vi "main.vi"() -> ()   [LabVIEW 2014]
uses:
  Step/Control/Step name enum.ctl
  Controls/Step array.ctl
  Controls/INI config.ctl
  <vilib>/DAQmx/read.llb/DAQmx Read (Analog DBL 1Chan 1Samp).vi
  <vilib>/Automated Test Systems Ltd/General Tools/Que lib/Initialise.vi
  <vilib>/Automated Test Systems Ltd/General Tools/Que lib/Write.vi
  <vilib>/DAQmx/miscellaneous.llb/DAQmx Fill In Error Info.vi
  Controls/ResultsGlobal.vi
  Controls/ConditionsGlobal.vi
  <vilib>/DAQmx/create/channels.llb/DAQmx Create Channel (AI-Temperature-Thermocouple).vi
  Step/Step global.vi
  Step/Test status global.vi
  <vilib>/Instr/_visa.llb/VISA Configure Serial Port (Instr).vi
  <vilib>/Automated Test Systems Ltd/Device drivers/SensorMetrix/Lib/Read T3110.vi
  <vilib>/NI/Modbus Library/API/Master/Modbus Master.lvclass
  <vilib>/Automated Test Systems Ltd/General Tools/Que lib/Que lib.lvlib
  <vilib>/Automated Test Systems Ltd/General Tools/Stopwatch/Stop watch/Stop watch.lvlib
  <vilib>/Automated Test Systems Ltd/Device drivers/SensorMetrix/Lib/T3110 & T2114.lvlib
panel:
  out "Test Status":string[](array[string])
  out "T3110 Temperature":dbl
  out "NI Temperature":dbl
  out "Arduino Temperature":dbl
  out "Step elapsed time, ms":u32
  out "Test elapsed time, ms":u32
  in  "pause":bool
  in  "abort":bool
  out "Step cluster":T2={"Step number"=0, "Step Name"="", "Step name enum"=enum."Init NI", "Start condition 1 name"="", "Start condition 1 comparator"="", "Start condition 1 value"=0.0, "Start condition 2 name"="", "Start condition 2 comparator"="", "Start condition 2 value"=0.0, "Start condition 3 name"="", "Start condition 3 comparator"="", "Start condition 3 value"=0.0, "End condition 1 name"="", "End condition 1 comparator"="", "End condition 1 value"=0.0, "End condition 2 name"="", "End condition 2 comparator"="", "End condition 2 value"=0.0, "End condition 3 name"="", "End condition 3 comparator"="", "End condition 3 value"=0.0, "Constant condition 1 name"="", "Constant condition 1 comparator"="", "Constant condition 1 value"=0.0, "Constant condition 2 name"="", "Constant condition 2 comparator"="", "Constant condition 2 value"=0.0, "Constant condition 3 name"="", "Constant condition 3 comparator"="", "Constant condition 3 value"=0.0, "Duration"=0.0, "Max Duration"=0.0}
  out "Test running":bool
  in  "file path (dialog if empty)":path
  in  "Start profile":bool
  out "Test profile INI":string[][](array[string])
  in  "stop":bool
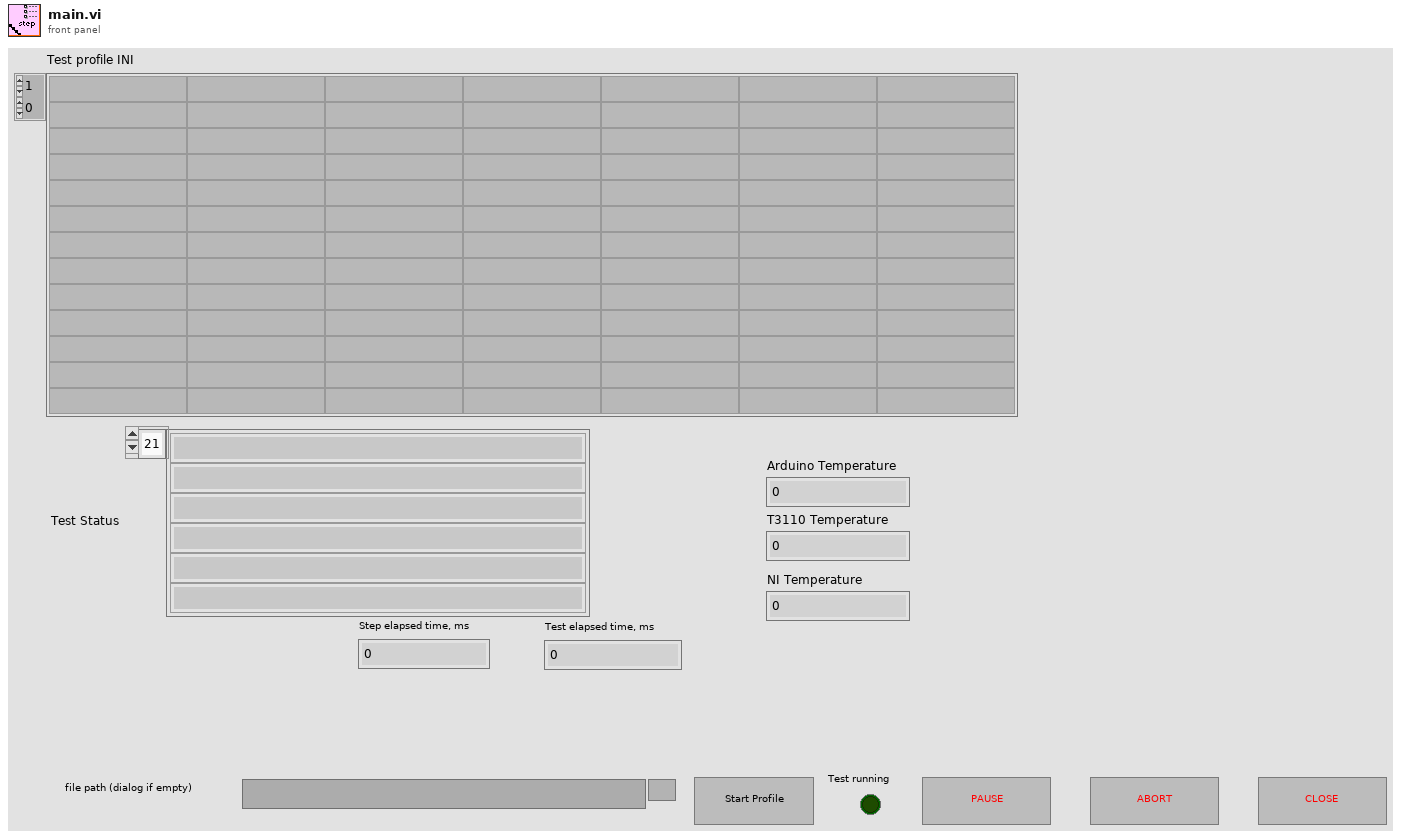
[diagram p1: front panel]
types:
  T1 = typedef "Step name enum.ctl" = enum16{"Default", "Idle", "Init Ard", "Init SM", "Init NI", "Run", "Close"}
  T2 = cluster{"Step number":i32, "Step Name":string, "Step name enum":T1, "Start condition 1 name":string, "Start condition 1 comparator":string, "Start condition 1 value":dbl, "Start condition 2 name":string, "Start condition 2 comparator":string, "Start condition 2 value":dbl, "Start condition 3 name":string, "Start condition 3 comparator":string, "Start condition 3 value":dbl, "End condition 1 name":string, "End condition 1 comparator":string, "End condition 1 value":dbl, "End condition 2 name":string, "End condition 2 comparator":string, "End condition 2 value":dbl, "End condition 3 name":string, "End condition 3 comparator":string, "End condition 3 value":dbl, "Constant condition 1 name":string, "Constant condition 1 comparator":string, "Constant condition 1 value":dbl, "Constant condition 2 name":string, "Constant condition 2 comparator":string, "Constant condition 2 value":dbl, "Constant condition 3 name":string, "Constant condition 3 comparator":string, "Constant condition 3 value":dbl, "Duration":dbl, "Max Duration":dbl}
  T3 = typedef "INI config.ctl" = cluster{"Config":cluster{"DAQ channel":string, "T3110 COM":string, "Arduino COM":string}, "Parameters":cluster{"Max temp":dbl, "Min temp":dbl}}
  T4 = typedef "Step array.ctl" = cluster{"Step number":i32, "Step Name":string, "Step name enum":T1, "Start condition 1 name":string, "Start condition 1 comparator":string, "Start condition 1 value":dbl, "Start condition 2 name":string, "Start condition 2 comparator":string, "Start condition 2 value":dbl, "Start condition 3 name":string, "Start condition 3 comparator":string, "Start condition 3 value":dbl, "End condition 1 name":string, "End condition 1 comparator":string, "End condition 1 value":dbl, "End condition 2 name":string, "End condition 2 comparator":string, "End condition 2 value":dbl, "End condition 3 name":string, "End condition 3 comparator":string, "End condition 3 value":dbl, "Constant condition 1 name":string, "Constant condition 1 comparator":string, "Constant condition 1 value":dbl, "Constant condition 2 name":string, "Constant condition 2 comparator":string, "Constant condition 2 value":dbl, "Constant condition 3 name":string, "Constant condition 3 comparator":string, "Constant condition 3 value":dbl, "Duration, mS":dbl, "Max Duration, mS":dbl}[]
  T5 = cluster{"Step number":i32, "Step Name":string, "Step name enum":T1, "Start condition 1 name":string, "Start condition 1 comparator":string, "Start condition 1 value":dbl, "Start condition 2 name":string, "Start condition 2 comparator":string, "Start condition 2 value":dbl, "Start condition 3 name":string, "Start condition 3 comparator":string, "Start condition 3 value":dbl, "End condition 1 name":string, "End condition 1 comparator":string, "End condition 1 value":dbl, "End condition 2 name":string, "End condition 2 comparator":string, "End condition 2 value":dbl, "End condition 3 name":string, "End condition 3 comparator":string, "End condition 3 value":dbl, "Constant condition 1 name":string, "Constant condition 1 comparator":string, "Constant condition 1 value":dbl, "Constant condition 2 name":string, "Constant condition 2 comparator":string, "Constant condition 2 value":dbl, "Constant condition 3 name":string, "Constant condition 3 comparator":string, "Constant condition 3 value":dbl, "Duration, mS":dbl, "Max Duration, mS":dbl}
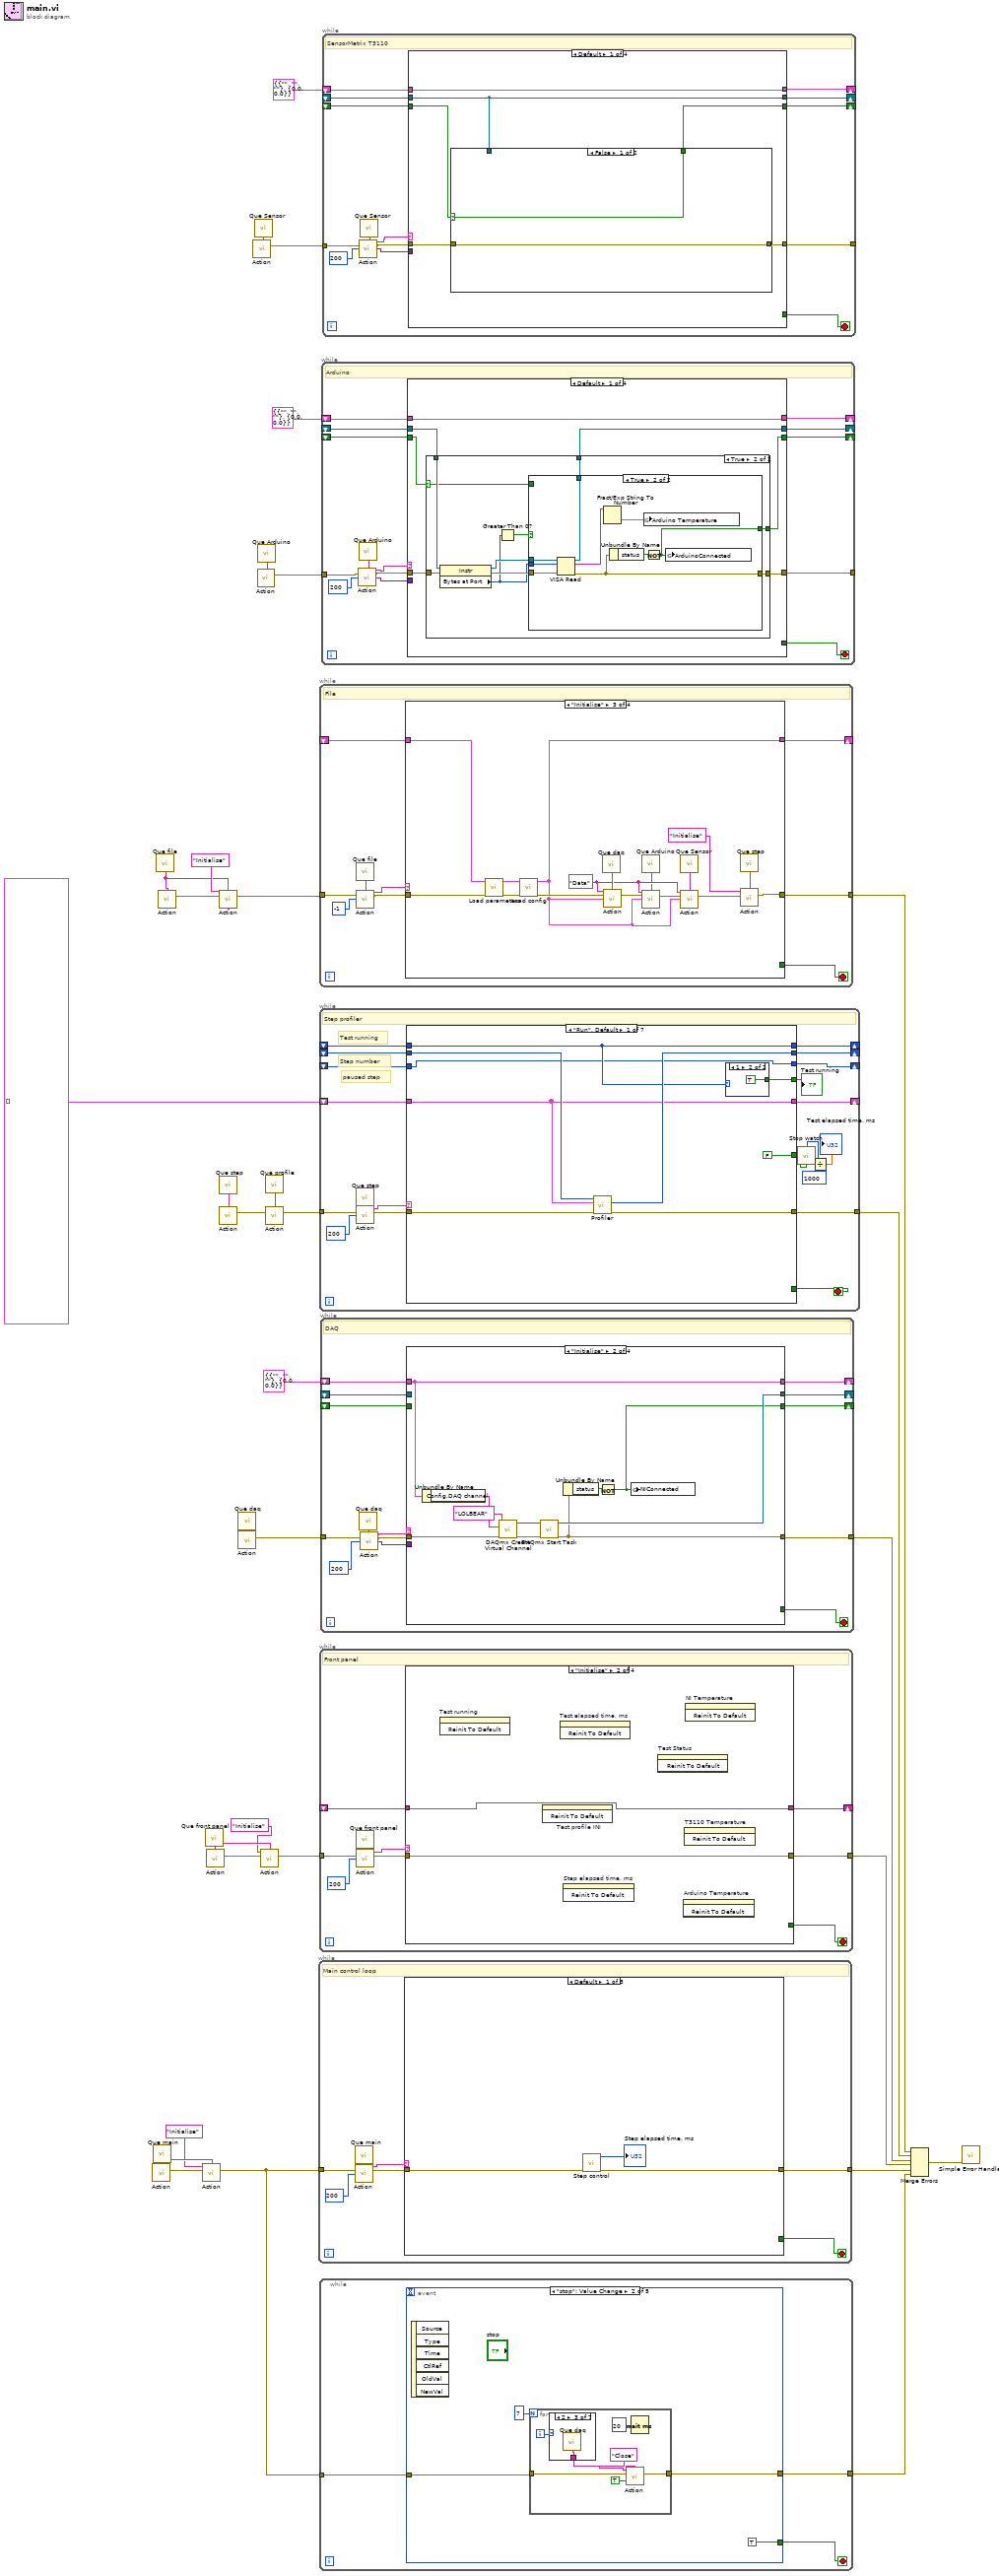
[diagram p0: block diagram]
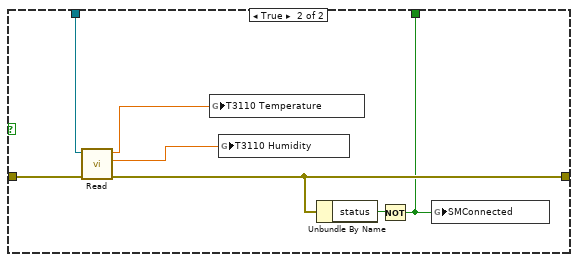
[diagram p2: hidden frame]
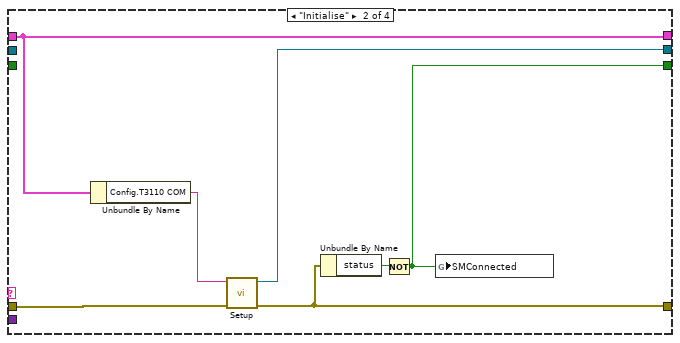
[diagram p3: hidden frame]
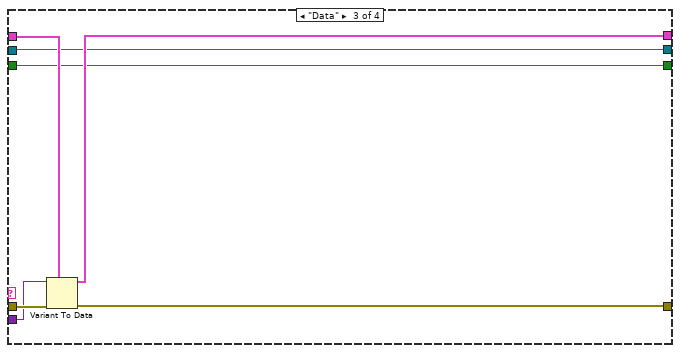
[diagram p4: hidden frame]
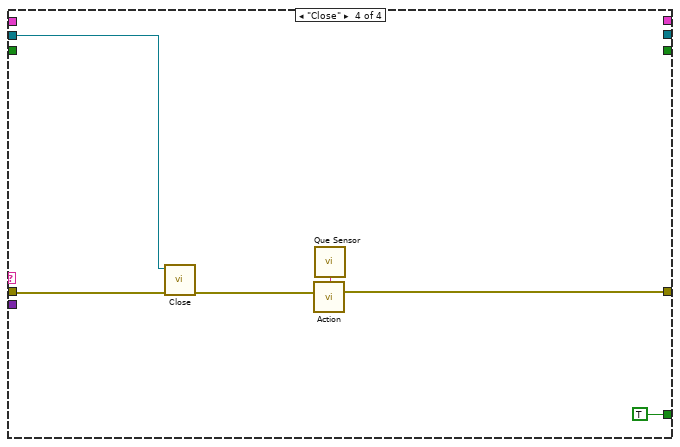
[diagram p5: hidden frame]
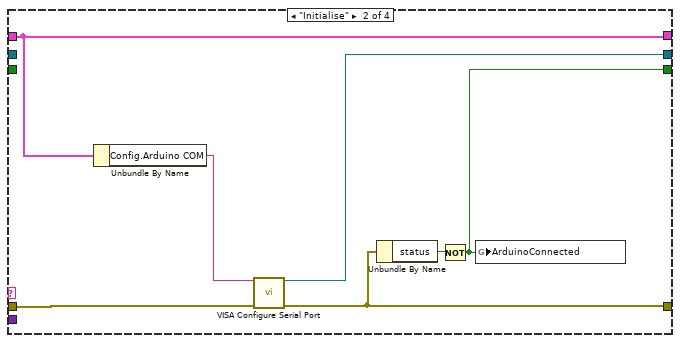
[diagram p8: hidden frame]
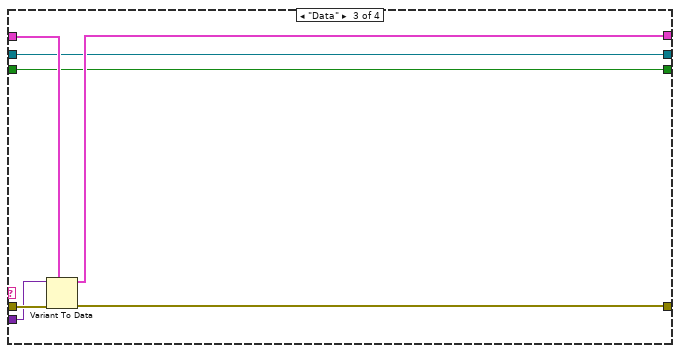
[diagram p9: hidden frame]
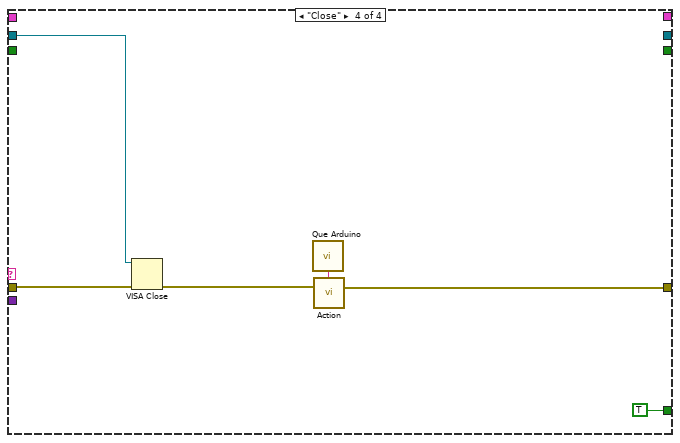
[diagram p10: hidden frame]
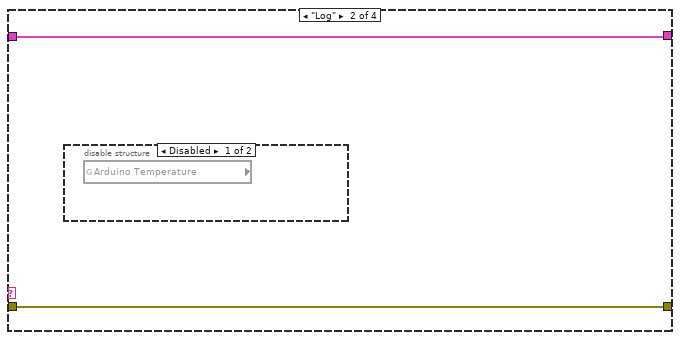
[diagram p12: hidden frame]
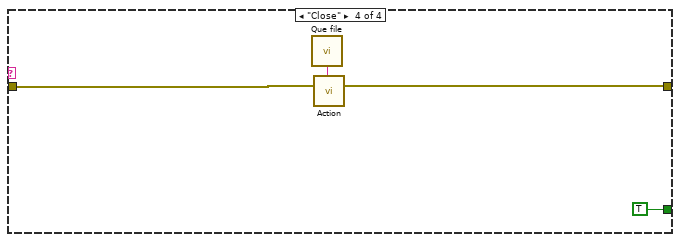
[diagram p14: hidden frame]
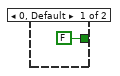
[diagram p15: hidden frame]
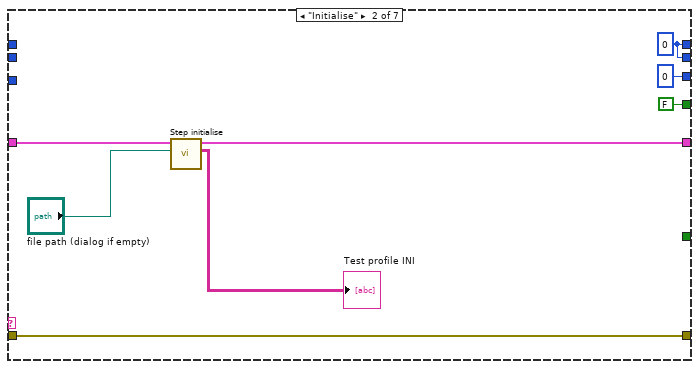
[diagram p16: hidden frame]
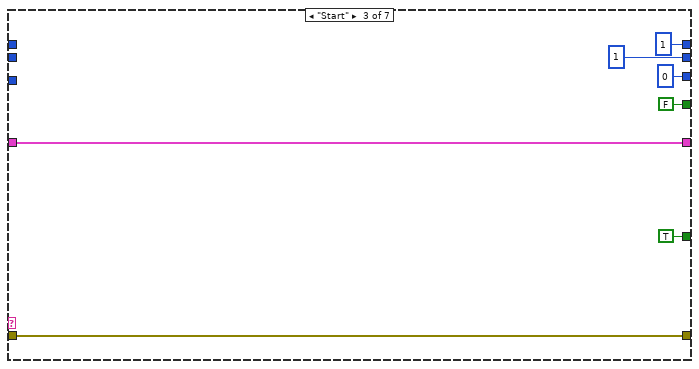
[diagram p17: hidden frame]
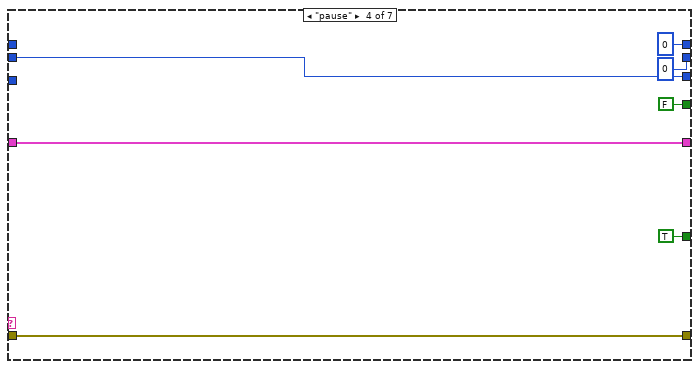
[diagram p18: hidden frame]
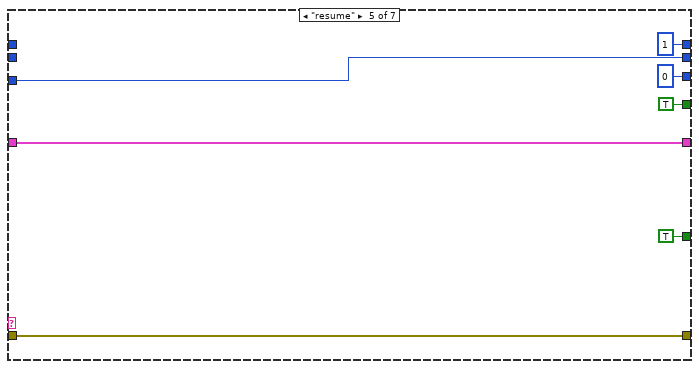
[diagram p19: hidden frame]
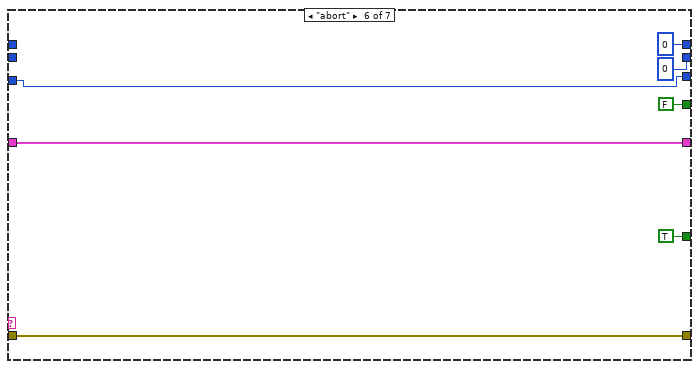
[diagram p20: hidden frame]
diagram:
  n1 = call <vilib>:"Que main.vi"() -> ("Que name"=w10:string)  [unwired: 15 in]
  n2 = call-poly <vilib>:"Action.vi"("Que name"=w10) -> ("error out"=w11:errorcluster)  [unwired: 14 in]
  n3 = call <vilib>:"Que file.vi"() -> ("Que name"=w22:string)  [unwired: 15 in]
  n4 = call-poly <vilib>:"Action.vi"("Que name"=w22) -> ("error out"=w23:errorcluster)  [unwired: 14 in]
  n5 = call-poly <vilib>:"Action.vi"("Message"="Initialise" ("Command"), "Que name"=w10, "error in"=w11) -> ("error out"=w8:errorcluster)  [unwired: 12 in]
  n6 = call <vilib>:"Que front panel.vi"() -> ("Que name"=w14:string)  [unwired: 15 in]
  n7 = call-poly <vilib>:"Action.vi"("Que name"=w14) -> ("error out"=w15:errorcluster)  [unwired: 14 in]
  n8 = call-poly <vilib>:"Action.vi"("Message"="Initialise" ("Command"), "Que name"=w22, "error in"=w23) -> ("error out"=w24:errorcluster)  [unwired: 12 in]
  n9 = call <vilib>:"Que step.vi"() -> ("Que name"=w18:string)  [unwired: 15 in]
  n10 = call-poly <vilib>:"Action.vi"("Que name"=w18) -> ("error out"=w21:errorcluster)  [unwired: 14 in]
  n11 = call <vilib>:"Que daq.vi"() -> ("Que name"=w17:string)  [unwired: 15 in]
  n12 = call-poly <vilib>:"Action.vi"("Que name"=w17) -> ("error out"=w16:errorcluster)  [unwired: 14 in]
  n13 = call <vilib>:"Que Sensor.vi"() -> ("Que name"=w4:string)  [unwired: 15 in]
  n14 = call-poly <vilib>:"Action.vi"("Que name"=w4) -> ("error out"=w3:errorcluster)  [unwired: 14 in]
  n15 = call <vilib>:"Que Arduino.vi"() -> ("Que name"=w6:string)  [unwired: 15 in]
  n16 = call-poly <vilib>:"Action.vi"("Que name"=w6) -> ("error out"=w7:errorcluster)  [unwired: 14 in]
  n17 = call-poly <vilib>:"Action.vi"("Message"="Initialise" ("Command"), "Que name"=w14, "error in"=w15) -> ("error out"=w13:errorcluster)  [unwired: 12 in]
  n18 = call <vilib>:"Que profile.vi"() -> ("Que name"=w19:string)  [unwired: 15 in]
  n19 = call-poly <vilib>:"Action.vi"("Que name"=w19, "error in"=w21) -> ("error out"=w20:errorcluster)  [unwired: 13 in]
  n20 = while {
    tunnel: w8 -> [w36]
    tunnel: [w40] -> w32
    stop <- w39 stop-if-true
    # "Main control loop"
    n21 = call <vilib>:"Que main.vi"() -> ("Que name"=w38:string)  [unwired: 15 in]
    n22 = call-poly <vilib>:"Action.vi"("Que name"=w38, "error in"=w36, "Timeout (default 2s)"=200 ("Timeout")) -> ("Message out"=w34:string, "error out"=w37:errorcluster)  [unwired: 10 in, 1 out]
    n23 = case shown="Default" w34 {
      tunnel: w37 -> [w43 w44 w46]
      tunnel: [w42 w44 w47] -> w40
      tunnel: [_ _ TRUE] -> w39
      frame Default {
        n24 = call "Step control.vi"("error in"=w43) -> ("error out"=w42:errorcluster, "Step elapsed time,  s"=→"Step elapsed time, ms":u32)  [unwired: 9 in]
      }
      frame "Initialise" {
      }
      frame "Close" {
        n25 = call <vilib>:"Que main.vi"() -> ("Que name"=w45:string)  [unwired: 15 in]
        n26 = call-poly <vilib>:"Action.vi"("Que name"=w45, "error in"=w46) -> ("error out"=w47:errorcluster)  [unwired: 13 in]
      }
    }
  }
  n27 = while {
    tunnel: w20 -> [w53]
    tunnel: [w67] -> w29
    shift-right: [w65] -> _
    shift-left: T4 [] ("Step array") -> [w66]
    shift-right: [w64] -> _
    shift-left: _ -> [w63]
    shift-right: [w61] -> _
    shift-left: _ -> [w62]
    shift-right: [w58] -> _
    shift-left: _ -> [w59]
    stop <- w68 stop-if-true
    # "paused step"
    # "Step number"
    # "Test running"
    # "Step profiler"
    n28 = call <vilib>:"Que step.vi"() -> ("Que name"=w51:string)  [unwired: 15 in]
    n29 = call-poly <vilib>:"Action.vi"("Que name"=w51, "error in"=w53, "Timeout (default 2s)"=200 ("Timeout")) -> ("Message out"=w54:string, "error out"=w55:errorcluster)  [unwired: 10 in, 1 out]
    n30 = case shown="\"Run\", Default" w54 {
      tunnel: w55 -> [w73 w87 w92 w99 w105 w112 w117]
      tunnel: [_ _ _ _ _ _ TRUE] -> w68
      tunnel: [w74 w87 w92 w99 w105 w112 w118] -> w67
      tunnel: w66 -> [w75 w85 w93 w96 w104 w113 w123]
      tunnel: [w75 w83 w93 w96 w104 w113 w123] -> w65
      tunnel: [w72 w86 1 0 1 0 0] -> w64
      tunnel: w63 -> [w72 _ _ _ _ _ _]
      tunnel: w62 -> [w77 _ _ w98 _ _ _]
      tunnel: [w76 w86 1 0 ("Step number") w107 0 ("Step number") 0] -> w61
      tunnel: [w70 FALSE FALSE FALSE TRUE FALSE FALSE] -> w60
      tunnel: w59 -> [w71 _ _ _ w107 w110 _]
      tunnel: [w71 0 ("Step number") 0 ("Step number") w98 0 ("Step number") w110 0 ("Step number")] -> w58
      tunnel: [FALSE _ TRUE TRUE TRUE TRUE _] -> w49
      frame "Run", Default {
        n31 = call "Profiler.vi"("error in"=w73, "Step array"=w75, "Step number"=w77) -> ("error out"=w74:errorcluster, "Step number"=w76:i32)  [unwired: 6 in, 1 out]
        n32 = case shown="1" w72 {
          tunnel: [FALSE TRUE] -> w70
          frame 0, Default {
          }
          frame 1 {
          }
        }
      }
      frame "Initialise" {
        w86 = 0
        n33 = call "Step initialise.vi"("file path (dialog if empty)"="file path (dialog if empty)", "Step array"=w85) -> ("all rows"=→"Test profile INI":string[][], "Step array out"=w83:T4)  [unwired: 8 in]
      }
      frame "Start" {
      }
      frame "pause" {
      }
      frame "resume" {
      }
      frame "abort" {
      }
      frame "Close" {
        n34 = call <vilib>:"Que step.vi"() -> ("Que name"=w116:string)  [unwired: 15 in]
        n35 = call-poly <vilib>:"Action.vi"("Que name"=w116, "error in"=w117) -> ("error out"=w118:errorcluster)  [unwired: 13 in]
      }
    }
    "Test running" <- w60
    n36 = call <vilib>:"Stop watch.vi"("reset timer"=w49) -> ("Elapsed time, ms"=w50:u32)  [unwired: 13 in, 1 out]
    n37 = Divide(x=w50, y=1000) -> (x/y=→"Test elapsed time, ms":dbl)
  }
  n38 = while {
    tunnel: w13 -> [w127]
    tunnel: [w132] -> w31
    shift-right: [w131] -> _
    shift-left: _ -> [w130]
    stop <- w133 stop-if-true
    # "Front panel"
    n39 = call <vilib>:"Que front panel.vi"() -> ("Que name"=w129:string)  [unwired: 15 in]
    n40 = call-poly <vilib>:"Action.vi"("Que name"=w129, "error in"=w127, "Timeout (default 2s)"=200 ("Timeout")) -> ("Message out"=w126:string, "error out"=w128:errorcluster)  [unwired: 10 in, 1 out]
    n41 = case shown="\"Initialise\"" w126 {
      tunnel: w128 -> [w142 w144 w146 w151]
      tunnel: [_ _ _ TRUE] -> w133
      tunnel: [w142 w144 w146 w148] -> w132
      tunnel: [w135 w143 w145 w150] -> w131
      tunnel: w130 -> [w140 w143 w145 w150]
      frame Default {
        n42 = global read "Step global.vi" "Step cluster"() -> (w141:T5)
        "Step cluster" <- w141
        n43 = global read "Test status global.vi" "Test status"() -> (w139:string)
        n44 = Unbundle(w141) -> ()  [unwired: 32 out]
        n45 = call <vilib>:"FILO string equal.vi"("Array"=w140, "Array size"=200, "String"=w139) -> ("Array out"=w135:string[])  [unwired: 12 in]
        "Test Status" <- w135
        n46 = global read "ResultsGlobal.vi" "Arduino Temperature"() -> (→"Arduino Temperature":dbl)
        n47 = global read "ResultsGlobal.vi" "T3110 Temperature"() -> (→"T3110 Temperature":dbl)
        n48 = global read "ResultsGlobal.vi" "NI Temperature"() -> (→"NI Temperature":dbl)
      }
      frame "Initialise" {
        n49 = invoke on="Test running" class="Bool (strict)" method="Reinit To Default"() -> ()  [unwired: 3 in, 3 out]
        n50 = invoke on="Test profile INI" class="Arr (strict)" method="Reinit To Default"() -> ()  [unwired: 3 in, 3 out]
        n51 = invoke on="Test elapsed time, ms" class="DigNum (strict)" method="Reinit To Default"() -> ()  [unwired: 3 in, 3 out]
        n52 = invoke on="Step elapsed time, ms" class="DigNum (strict)" method="Reinit To Default"() -> ()  [unwired: 3 in, 3 out]
        n53 = invoke on="Test Status" class="Arr (strict)" method="Reinit To Default"() -> ()  [unwired: 3 in, 3 out]
        n54 = invoke on="Arduino Temperature" class="DigNum (strict)" method="Reinit To Default"() -> ()  [unwired: 3 in, 3 out]
        n55 = invoke on="T3110 Temperature" class="DigNum (strict)" method="Reinit To Default"() -> ()  [unwired: 3 in, 3 out]
        n56 = invoke on="NI Temperature" class="DigNum (strict)" method="Reinit To Default"() -> ()  [unwired: 3 in, 3 out]
      }
      frame "clear" {
      }
      frame "Close" {
        n57 = invoke on="Test profile INI" class="Arr (strict)" method="Reinit To Default"(error in=w151) -> (error out=w149:errorcluster)  [unwired: 2 in, 2 out]
        n58 = call <vilib>:"Que front panel.vi"() -> ("Que name"=w147:string)  [unwired: 15 in]
        n59 = call-poly <vilib>:"Action.vi"("Que name"=w147, "error in"=w149) -> ("error out"=w148:errorcluster)  [unwired: 13 in]
      }
    }
  }
  n60 = while {
    tunnel: w8 -> [w155]
    tunnel: [w154] -> w33
    stop <- w153 stop-if-true
    n61 = event shown="[1] \"stop\": Value Change" {
      selector: _ -> [_ _ _ _ _]
      dyn-events: _ -> [_ _ _ _ _]
      timeout: _ -> [_ _ _ _ _]
      tunnel: w155 -> [_ w158 w176 w180 w184]
      tunnel: [_ w157 w178 w181 w185] -> w154
      tunnel: [_ TRUE _ _ _] -> w153
      event Timeout {
        n62 = event-data() -> ()  [unwired: 1 in, 2 out]
      }
      event "stop": Value Change {
        n63 = event-data() -> ()  [unwired: 1 in, 6 out]
        n64 = for {
          N: 7 -> [_]
          tunnel: w158 -> [w162]
          tunnel: [w163] -> w157
          i -> [w166]
          n65 = case shown="2" w166 {
            tunnel: [w167 w168 w169 w170 w171 w172 w173] -> w160
            frame 0, Default {
              n66 = call <vilib>:"Que file.vi"() -> ("Que name"=w167:string)  [unwired: 15 in]
            }
            frame 1 {
              n67 = call <vilib>:"Que front panel.vi"() -> ("Que name"=w168:string)  [unwired: 15 in]
            }
            frame 2 {
              n68 = call <vilib>:"Que daq.vi"() -> ("Que name"=w169:string)  [unwired: 15 in]
            }
            frame 3 {
              n69 = call <vilib>:"Que main.vi"() -> ("Que name"=w170:string)  [unwired: 15 in]
            }
            frame 4 {
              n70 = call <vilib>:"Que step.vi"() -> ("Que name"=w171:string)  [unwired: 15 in]
            }
            frame 5 {
              n71 = call <vilib>:"Que Arduino.vi"() -> ("Que name"=w172:string)  [unwired: 15 in]
            }
            frame 6 {
              n72 = call <vilib>:"Que Sensor.vi"() -> ("Que name"=w173:string)  [unwired: 15 in]
            }
          }
          n73 = call-poly <vilib>:"Action.vi"("Message"="Close" ("Command"), "Que name"=w160, "error in"=w162, "Priority message?"=TRUE) -> ("error out"=w163:errorcluster)  [unwired: 11 in]
          n74 = Wait (ms)(milliseconds to wait=u32 20) -> ()  [unwired: 1 out]
        }
      }
      event "abort": Value Change {
        n75 = event-data() -> ()  [unwired: 1 in, 6 out]
        n76 = call <vilib>:"Que step.vi"() -> ("Que name"=w177:string)  [unwired: 15 in]
        n77 = call-poly <vilib>:"Action.vi"("Message"="abort" ("Command"), "Que name"=w177, "error in"=w176, "Priority message?"=TRUE) -> ("error out"=w178:errorcluster)  [unwired: 11 in]
      }
      event "Start profile": Value Change {
        n78 = event-data() -> ()  [unwired: 1 in, 6 out]
        n79 = call <vilib>:"Que step.vi"() -> ("Que name"=w182:string)  [unwired: 15 in]
        n80 = call-poly <vilib>:"Action.vi"("Message"="Start" ("Command"), "Que name"=w182, "error in"=w180) -> ("error out"=w181:errorcluster)  [unwired: 12 in]
      }
      event "pause": Value Change {
        n81 = event-data() -> ()  [unwired: 1 in, 6 out]
        n82 = case shown="False" "pause" {
          tunnel: ["resume" ("Command") "pause" ("Command")] -> w183
          tunnel: ["PAUSE" ("Command") "RESUME" ("Command")] -> w187
          frame False {
          }
          frame True {
          }
        }
        n83 = property on="pause" class="Bool (strict)"("BoolText.Text"=w187) -> ()  [unwired: 2 in, 2 out]
        n84 = call <vilib>:"Que step.vi"() -> ("Que name"=w186:string)  [unwired: 15 in]
        n85 = call-poly <vilib>:"Action.vi"("Message"=w183, "Que name"=w186, "error in"=w184) -> ("error out"=w185:errorcluster)  [unwired: 12 in]
      }
    }
  }
  n86 = while {
    tunnel: w24 -> [w199]
    tunnel: [w200] -> w28
    shift-right: [w194] -> _
    shift-left: _ -> [w193]
    stop <- w201 stop-if-true
    # "File"
    n87 = call <vilib>:"Que file.vi"() -> ("Que name"=w195:string)  [unwired: 15 in]
    n88 = call-poly <vilib>:"Action.vi"("Que name"=w195, "error in"=w199, "Timeout (default 2s)"=-1 ("Timeout")) -> ("Message out"=w197:string, "error out"=w198:errorcluster)  [unwired: 10 in, 1 out]
    n89 = case shown="\"Initialise\"" w197 {
      tunnel: w198 -> [w203 w205 w218 w224]
      tunnel: [_ _ _ TRUE] -> w201
      tunnel: [w203 w205 w221 w223] -> w200
      tunnel: [w202 w204 w211 _] -> w194
      tunnel: w193 -> [w202 w204 w214 _]
      frame Default {
      }
      frame "Log" {
        n90 = disable-structure shown="Disabled" {
          frame Disabled {
            n91 = global read "ResultsGlobal.vi" "Arduino Temperature"() -> ()  [unwired: 1 out]
          }
          frame Enabled {
          }
        }
      }
      frame "Initialise" {
        w210 = "Data" ("Command")
        n92 = call "Load parameters.vi"("error in"=w218, "INI data"=w214) -> ("error out"=w217:errorcluster, "INI data out"=w215:T3)  [unwired: 8 in]
        n93 = call "Load config.vi"("error in"=w217, "INI data"=w215) -> ("error out"=w216:errorcluster, "INI data out"=w211:T3)  [unwired: 8 in]
        n94 = call <vilib>:"Que daq.vi"() -> ("Que name"=w219:string)  [unwired: 15 in]
        n95 = call-poly <vilib>:"Action.vi"("Message"=w210, "Que name"=w219, "error in"=w216, "Data"=w211) -> ("error out"=w213:errorcluster)  [unwired: 11 in]
        n96 = call <vilib>:"Que Arduino.vi"() -> ("Que name"=w208:string)  [unwired: 15 in]
        n97 = call-poly <vilib>:"Action.vi"("Message"=w210, "Que name"=w208, "error in"=w213, "Data"=w211) -> ("error out"=w212:errorcluster)  [unwired: 11 in]
        n98 = call <vilib>:"Que Sensor.vi"() -> ("Que name"=w209:string)  [unwired: 15 in]
        n99 = call-poly <vilib>:"Action.vi"("Message"=w210, "Que name"=w209, "error in"=w212, "Data"=w211) -> ("error out"=w207:errorcluster)  [unwired: 11 in]
        n100 = call <vilib>:"Que step.vi"() -> ("Que name"=w220:string)  [unwired: 15 in]
        n101 = call-poly <vilib>:"Action.vi"("Message"="Initialise" ("Command"), "Que name"=w220, "error in"=w207) -> ("error out"=w221:errorcluster)  [unwired: 12 in]
      }
      frame "Close" {
        n102 = call <vilib>:"Que file.vi"() -> ("Que name"=w222:string)  [unwired: 15 in]
        n103 = call-poly <vilib>:"Action.vi"("Que name"=w222, "error in"=w224) -> ("error out"=w223:errorcluster)  [unwired: 13 in]
      }
    }
  }
  n104 = while {
    tunnel: w16 -> [w236]
    tunnel: [w238] -> w30
    shift-right: [w231] -> _
    shift-left: T3 {"Config"={"DAQ channel"="", "T3110 COM"="", "Arduino COM"=""}, "Parameters"={"Max temp"=0.0, "Min temp"=0.0}} ("INI data") -> [w230]
    shift-right: [w229] -> _
    shift-left: _ -> [w228]
    shift-right: [w227] -> _
    shift-left: _ -> [w226]
    stop <- w239 stop-if-true
    # "DAQ"
    n105 = call <vilib>:"Que daq.vi"() -> ("Que name"=w237:string)  [unwired: 15 in]
    n106 = call-poly <vilib>:"Action.vi"("Que name"=w237, "error in"=w236, "Timeout (default 2s)"=200 ("Timeout")) -> ("Message out"=w234:string, "error out"=w235:errorcluster, "Data"=w232:variant)  [unwired: 10 in]
    n107 = case shown="\"Initialise\"" w234 {
      tunnel: w235 -> [w244 w259 w271 w274]
      tunnel: [_ _ _ TRUE] -> w239
      tunnel: [w243 w258 w267 w278] -> w238
      tunnel: w232 -> [_ _ w270 _]
      tunnel: w230 -> [w245 w260 w269 _]
      tunnel: [w245 w260 w268 _] -> w231
      tunnel: [w242 w261 w266 _] -> w229
      tunnel: w228 -> [w242 _ w266 w272]
      tunnel: [w240 w256 w265 _] -> w227
      tunnel: w226 -> [w241 _ w265 _]
      frame Default {
        n108 = case shown="True" w241 {
          selector: w241 -> [w247 _]
          tunnel: w244 -> [w246 w254]
          tunnel: [w246 w251] -> w243
          tunnel: w242 -> [_ w253]
          tunnel: [w247 w250] -> w240
          frame False {
          }
          frame True {
            n109 = call-poly <vilib>:"DAQmx Read.vi"("task/channels in"=w253, "error in"=w254) -> ("data"=w248:dbl, "error out"=w251:errorcluster)  [unwired: 11 in, 1 out]
            n110 = To Double Precision Float(number=w248) -> (double precision float=w249:dbl)
            n111 = global write "ResultsGlobal.vi" "NI Temperature"(w249) -> ()
            n112 = Unbundle By Name(w251) -> ("status"=w252:bool)
            n113 = Not(x=w252) -> (.not. x?=w250:bool)
            n114 = global write "ConditionsGlobal.vi" "NIConnected"(w250) -> ()
          }
        }
      }
      frame "Initialise" {
        n115 = Unbundle By Name(w260) -> ("Config.DAQ channel"=w263:string)
        n116 = call-poly <vilib>:"DAQmx Create Virtual Channel.vi"("physical channels"=w263, "name to assign"="LOLBEAR", "error in"=w259) -> ("task out"=w262:refnum<k21>, "error out"=w264:errorcluster)  [unwired: 11 in]
        n117 = call <vilib>:"DAQmx Start Task.vi"("task/channels in"=w262, "error in"=w264) -> ("task out"=w261:refnum<k21>, "error out"=w258:errorcluster)  [unwired: 12 in]
        n118 = Unbundle By Name(w258) -> ("status"=w257:bool)
        n119 = Not(x=w257) -> (.not. x?=w256:bool)
        n120 = global write "ConditionsGlobal.vi" "NIConnected"(w256) -> ()
      }
      frame "Data" {
        n121 = Variant To Data(error in=w271, type=w269, Variant=w270) -> (data=w268:T3, error out=w267:errorcluster)
      }
      frame "Close" {
        n122 = call <vilib>:"DAQmx Stop Task.vi"("task/channels in"=w272, "error in"=w274) -> ("task out"=w273:refnum<k21>, "error out"=w275:errorcluster)  [unwired: 12 in]
        n123 = call <vilib>:"DAQmx Clear Task.vi"("task in"=w273, "error in"=w275) -> ("error out"=w276:errorcluster)  [unwired: 13 in]
        n124 = call <vilib>:"Que daq.vi"() -> ("Que name"=w277:string)  [unwired: 15 in]
        n125 = call-poly <vilib>:"Action.vi"("Que name"=w277, "error in"=w276) -> ("error out"=w278:errorcluster)  [unwired: 13 in]
      }
    }
  }
  n126 = while {
    tunnel: [w292] -> _
    shift-right: [w288] -> _
    shift-left: T3 {"Config"={"DAQ channel"="", "T3110 COM"="", "Arduino COM"=""}, "Parameters"={"Max temp"=0.0, "Min temp"=0.0}} ("INI data") -> [w287]
    tunnel: w7 -> [w285]
    shift-right: [w283] -> _
    shift-left: _ -> [w282]
    shift-right: [w281] -> _
    shift-left: _ -> [w280]
    stop <- w293 stop-if-true
    # "Arduino"
    n127 = call <vilib>:"Que Arduino.vi"() -> ("Que name"=w286:string)  [unwired: 15 in]
    n128 = call-poly <vilib>:"Action.vi"("Que name"=w286, "error in"=w285, "Timeout (default 2s)"=200 ("Timeout")) -> ("Message out"=w290:string, "error out"=w291:errorcluster, "Data"=w284:variant)  [unwired: 10 in]
    n129 = case shown="Default" w290 {
      tunnel: w291 -> [w297 w330 w339 w342]
      tunnel: [_ _ _ TRUE] -> w293
      tunnel: [w298 w327 w335 w344] -> w292
      tunnel: [w300 w329 w336 _] -> w288
      tunnel: w287 -> [w300 w329 w337 _]
      tunnel: w284 -> [_ _ w338 _]
      tunnel: [w299 w332 w334 _] -> w283
      tunnel: w282 -> [w296 _ w334 w340]
      tunnel: [w294 w326 w333 _] -> w281
      tunnel: w280 -> [w295 _ w333 _]
      frame Default {
        n130 = case shown="True" w295 {
          selector: w295 -> [w301 w304]
          tunnel: [w302 w313] -> w299
          tunnel: [w303 w312] -> w298
          tunnel: w297 -> [w303 w311]
          tunnel: w296 -> [w302 w310]
          tunnel: [w301 w305] -> w294
          frame False {
          }
          frame True {
            n131 = property class="Instr"(reference=w310, error in=w311) -> (reference out=w309:refnum<visa-resource-name>, error out=w308:errorcluster, "Bytes at Port"=w307:u32)
            n132 = Greater Than 0?(x=w307) -> (x > 0?=w306:bool)
            n133 = case shown="True" w306 {
              tunnel: [w315 w325] -> w313
              tunnel: [w316 w318] -> w312
              tunnel: w309 -> [w315 w324]
              tunnel: w308 -> [w316 w323]
              tunnel: w307 -> [_ w322]
              tunnel: [w314 w317] -> w305
              tunnel: w304 -> [w314 _]
              frame False {
              }
              frame True {
                n134 = VISA Read(VISA resource name=w324, byte count=w322, error in (no error)=w323) -> (VISA resource name out=w325:refnum<visa-resource-name>, read buffer=w321:string, error out=w318:errorcluster)  [unwired: 1 out]
                n135 = Fract/Exp String To Number(string=w321) -> (number=w320:dbl)  [unwired: 3 in, 1 out]
                n136 = Unbundle By Name(w318) -> ("status"=w319:bool)
                n137 = global write "ResultsGlobal.vi" "Arduino Temperature"(w320) -> ()
                n138 = Not(x=w319) -> (.not. x?=w317:bool)
                n139 = global write "ConditionsGlobal.vi" "ArduinoConnected"(w317) -> ()
              }
            }
          }
        }
      }
      frame "Initialise" {
        n140 = Unbundle By Name(w329) -> ("Config.Arduino COM"=w331:string)
        n141 = call-poly "VISA Configure Serial Port"("VISA resource name"=w331, "error in (no error)"=w330) -> ("VISA resource name out"=w332:refnum<visa-resource-name>, "error out"=w327:errorcluster)  [unwired: 12 in]
        n142 = Unbundle By Name(w327) -> ("status"=w328:bool)
        n143 = Not(x=w328) -> (.not. x?=w326:bool)
        n144 = global write "ConditionsGlobal.vi" "ArduinoConnected"(w326) -> ()
      }
      frame "Data" {
        n145 = Variant To Data(error in=w339, type=w337, Variant=w338) -> (data=w336:T3, error out=w335:errorcluster)
      }
      frame "Close" {
        n146 = VISA Close(VISA resource name=w340, error in (no error)=w342) -> (error out=w341:errorcluster)
        n147 = call <vilib>:"Que Arduino.vi"() -> ("Que name"=w343:string)  [unwired: 15 in]
        n148 = call-poly <vilib>:"Action.vi"("Que name"=w343, "error in"=w341) -> ("error out"=w344:errorcluster)  [unwired: 13 in]
      }
    }
  }
  n149 = while {
    tunnel: [w358] -> _
    shift-right: [w354] -> _
    shift-left: T3 {"Config"={"DAQ channel"="", "T3110 COM"="", "Arduino COM"=""}, "Parameters"={"Max temp"=0.0, "Min temp"=0.0}} ("INI data") -> [w353]
    tunnel: w3 -> [w352]
    shift-right: [w349] -> _
    shift-left: _ -> [w348]
    shift-right: [w347] -> _
    shift-left: _ -> [w346]
    stop <- w359 stop-if-true
    # "SensorMetrix T3110"
    n150 = call <vilib>:"Que Sensor.vi"() -> ("Que name"=w350:string)  [unwired: 15 in]
    n151 = call-poly <vilib>:"Action.vi"("Que name"=w350, "error in"=w352, "Timeout (default 2s)"=200 ("Timeout")) -> ("Message out"=w356:string, "error out"=w357:errorcluster, "Data"=w351:variant)  [unwired: 10 in]
    n152 = case shown="Default" w356 {
      tunnel: w357 -> [w364 w378 w388 w390]
      tunnel: [_ _ _ TRUE] -> w359
      tunnel: [w363 w376 w384 w393] -> w358
      tunnel: [w365 w379 w385 _] -> w354
      tunnel: w353 -> [w365 w379 w386 _]
      tunnel: w351 -> [_ _ w387 _]
      tunnel: [w362 w380 w383 _] -> w349
      tunnel: w348 -> [w362 _ w383 w389]
      tunnel: [w361 w375 w382 _] -> w347
      tunnel: w346 -> [w360 _ w382 _]
      frame Default {
        n153 = case shown="False" w360 {
          selector: w360 -> [w366 _]
          tunnel: w364 -> [w367 w374]
          tunnel: [w367 w369] -> w363
          tunnel: w362 -> [_ w372]
          tunnel: [w366 w368] -> w361
          frame False {
          }
          frame True {
            n154 = call-poly <vilib>:"Read.vi"("error in"=w374, "Modbus master in"=w372) -> ("error out"=w369:errorcluster, "Humidity, %"=w371:dbl, "Temperature, deg C"=w373:dbl)  [unwired: 7 in]
            n155 = global write "ResultsGlobal.vi" "T3110 Temperature"(w373) -> ()
            n156 = global write "ResultsGlobal.vi" "T3110 Humidity"(w371) -> ()
            n157 = Unbundle By Name(w369) -> ("status"=w370:bool)
            n158 = Not(x=w370) -> (.not. x?=w368:bool)
            n159 = global write "ConditionsGlobal.vi" "SMConnected"(w368) -> ()
          }
        }
      }
      frame "Initialise" {
        n160 = Unbundle By Name(w379) -> ("Config.T3110 COM"=w381:string)
        n161 = call <vilib>:"Setup.vi"("error in"=w378, "Sensormetrix COM port"=w381) -> ("error out"=w376:errorcluster, "Modbus master out"=w380:refnum<class "Modbus Master.lvclass">)  [unwired: 8 in]
        n162 = Unbundle By Name(w376) -> ("status"=w377:bool)
        n163 = Not(x=w377) -> (.not. x?=w375:bool)
        n164 = global write "ConditionsGlobal.vi" "SMConnected"(w375) -> ()
      }
      frame "Data" {
        n165 = Variant To Data(error in=w388, type=w386, Variant=w387) -> (data=w385:T3, error out=w384:errorcluster)
      }
      frame "Close" {
        n166 = call <vilib>:"Close.vi"("error in"=w390, "Modbus instance in"=w389) -> ("error out"=w391:errorcluster)  [unwired: 9 in]
        n167 = call <vilib>:"Que Sensor.vi"() -> ("Que name"=w392:string)  [unwired: 15 in]
        n168 = call-poly <vilib>:"Action.vi"("Que name"=w392, "error in"=w391) -> ("error out"=w393:errorcluster)  [unwired: 13 in]
      }
    }
  }
  n169 = Merge Errors(w28, w29, w30, w31, w32, w33) -> (w27:errorcluster)
  n170 = call <vilib>:"Simple Error Handler.vi"("error in (no error)"=w27) -> ()  [unwired: 4 in, 5 out]
